vi "Test Find Tests From Directory.vi"(8 "error in (no error)":errorcluster, 11 "Test Case In":refnum<class "Test FInder Test.lvclass">) -> (0 "error out":errorcluster, 3 "Test Case Out":refnum<class "Test FInder Test.lvclass">)   [LabVIEW 2020, in "Test FInder Test.lvclass"]
uses:
  Test FInder Test.lvclass
  C:/Program Files (x86)/National Instruments/LabVIEW 2020/vi.lib/Astemes/LUnit/Test Case.lvclass
  <vilib>/Astemes/LUnit/Test Case.lvclass/Test Case.ctl
  251402f5-1280-4c2e-a1c6-c7b73fef075a.vi
  <vilib>/Astemes/LUnit/Palette/Pass If.vi
  <vilib>/Astemes/LUnit/Core/LUnit Test Case/Private/Append Fail Result.vi
  <vilib>/Astemes/LUnit/Core/LUnit Test Case/Private/Append Pass Result.vi
  <vilib>/Astemes/LUnit/Core/LUnit Test Case/Private/Run In UI.vi
  <vilib>/Utility/error.llb/Clear Errors.vi
  source/Framework/Test Finder/Test Finder.lvclass
  source/LUnit Test Suite.lvclass
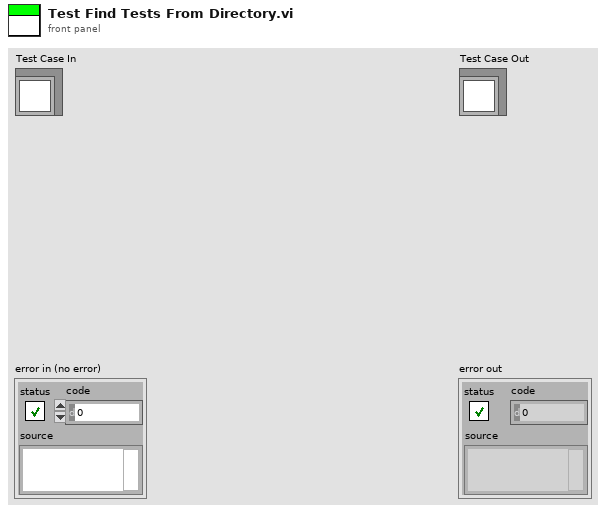
[diagram p1: front panel]
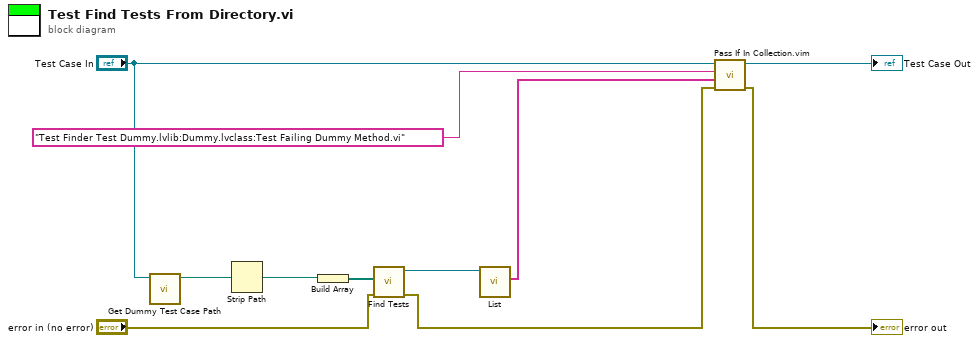
[diagram p0: block diagram]
diagram:
  n1 = call "Get Dummy Test Case Path.vi"("LUnit Test Suite Tests in"="Test Case In") -> ("appended path"=w8:path)  [unwired: 10 in]
  n2 = Strip Path(path=w8) -> (stripped path=w2:path)  [unwired: 1 out]
  n3 = Build Array(w2) -> (w7:path[])
  n4 = call "Find Tests.vi"("error in (no error)"="error in (no error)", "File Paths"=w7) -> ("error out"=w9:errorcluster, "LUnit Test Suite"=w6:refnum<class "LUnit Test Suite.lvclass">)  [unwired: 8 in]
  n5 = call "List.vi"("LUnit Test Suite In"=w6) -> ("List of Runnables"=w5:string[])  [unwired: 9 in, 1 out]
  n6 = call "Pass If In Collection.vim"("error in (no error)"=w9, "Collection"=w5, "Expected Element"="Test Finder Test Dummy.lvlib:Dummy.lvclass:Test Failing Dummy Method.vi" ("format string"), "LUnit Test Case In"="Test Case In") -> ("error out"=→"error out":errorcluster, "LUnit Test Case Out"=→"Test Case Out":refnum<class "Test FInder Test.lvclass">)  [unwired: 6 in]
